vi "Read.vi"(8 "error in (no error)":errorcluster, 11 "Boolean Array in":refnum<class "Boolean Array.lvclass">) -> (0 "error out":errorcluster, 2 "Boolean Array":bool[](array[boolean]), 3 "Boolean Array out":refnum<class "Boolean Array.lvclass">)   [LabVIEW 2020, in "Data.lvlib" / "Boolean Array.lvclass"]
doc: "Read Boolean Array."
uses:
  Boolean Array.lvclass
  Boolean Array.lvclass/Boolean Array.ctl
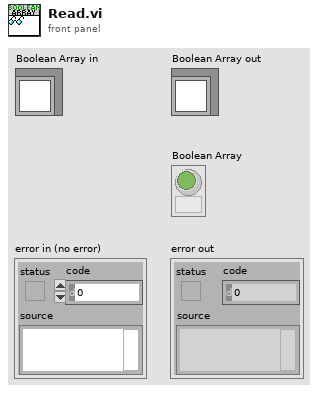
[diagram p1: front panel]
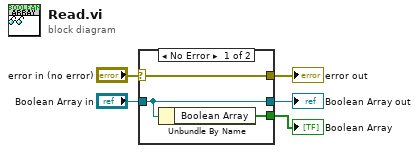
[diagram p0: block diagram]
diagram:
  n1 = case shown="No Error" "error in (no error)" {
    selector: "error in (no error)" -> [w8 w9]
    tunnel: [w8 w9] -> w4
    tunnel: [w7 w10] -> w2
    tunnel: "Boolean Array in" -> [w7 w10]
    tunnel: [w6 _] -> w1
    frame No Error {
      n2 = Unbundle By Name(w7) -> ("Boolean Array"=w6:bool[])
    }
    frame Error {
    }
  }
  "error out" <- w4
  "Boolean Array out" <- w2
  "Boolean Array" <- w1
